vi "Test ARINC API.vi"() -> ()   [LabVIEW 2021]
doc: "ARINC API Tester."
uses:
  <vilib>/Utility/miscctls.llb/LVPointTypeDef.ctl
  <vilib>/Utility/error.llb/DialogType.ctl
  ARINC.lvlib
panel:
  in  "REQ Close Ref":bool
  out "Connect?":bool
  in  "serial number":u64
  in  "DAQ Type":enum16{"Hardware", "Simulation"}(ring)
  in  "REQ Initialize Hardware":bool
  in  "Show Diagram on Init":bool
  in  "Show Block Diagram":bool
  in  "Stop Module":bool
  in  "Start Module":bool
  in  "Hide Module Panel":bool
  in  "Show Module Panel":bool
  out "Status":string
  out "Module Running?":bool
  # "This VI tests the API for the Module."
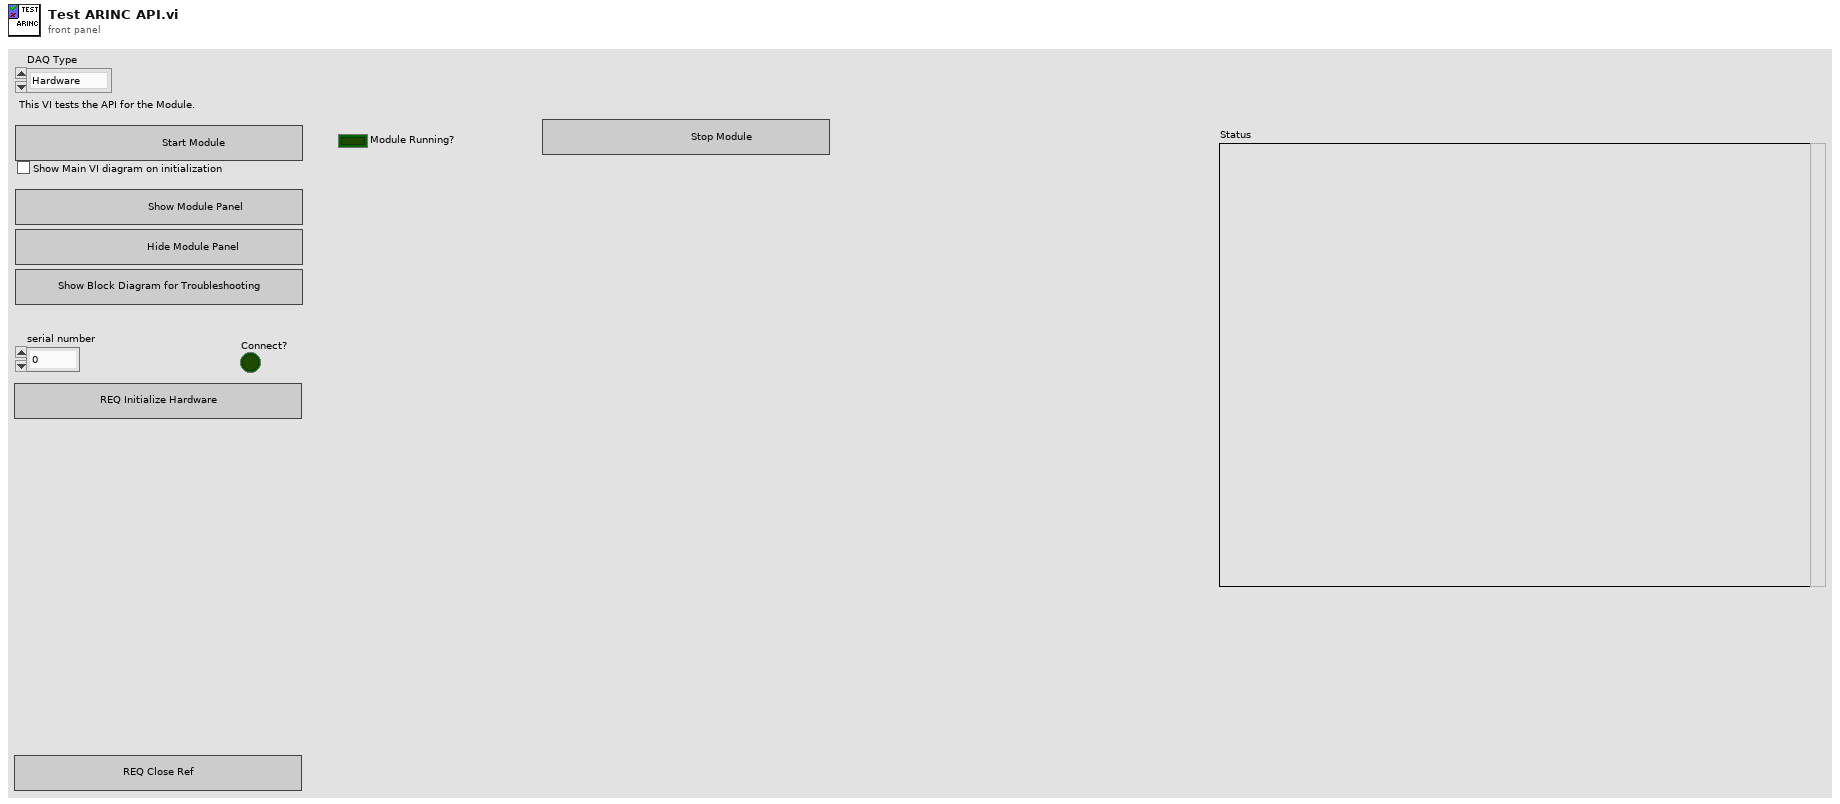
[diagram p1: front panel]
types:
  T1 = typedef "LVPointTypeDef.ctl" = cluster{"Horizontal":i16, "Vertical":i16}
  T2 = typedef "ARINC.lvlib/Broadcast Events--cluster.ctl" = cluster{"Module Did Init":refnum<user-event>, "Status Updated":refnum<user-event>, "Error Reported":refnum<user-event>, "Module Did Stop":refnum<user-event>, "Update Module Execution Status":refnum<user-event>}
  T3 = typedef "DialogType.ctl" = u16
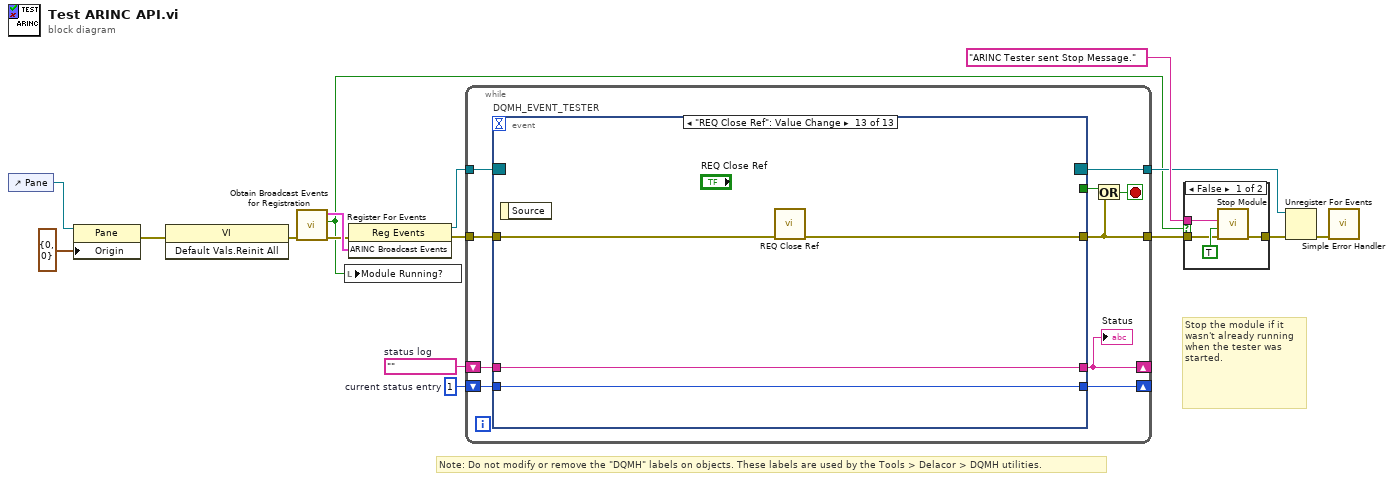
[diagram p0: block diagram]
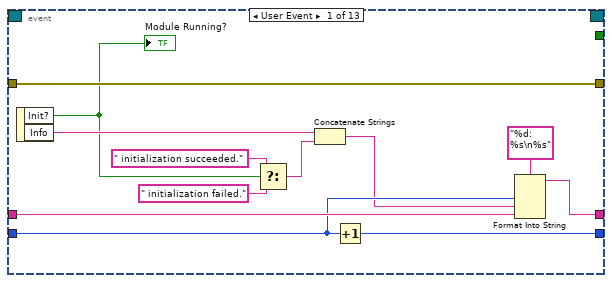
[diagram p3: hidden frame]
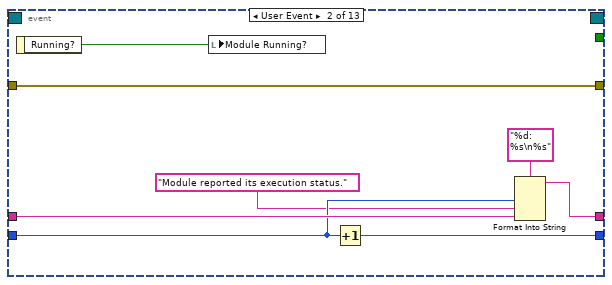
[diagram p4: hidden frame]
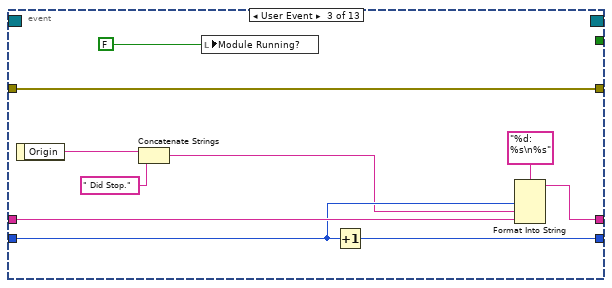
[diagram p5: hidden frame]
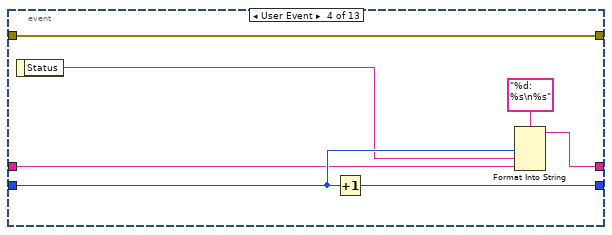
[diagram p6: hidden frame]
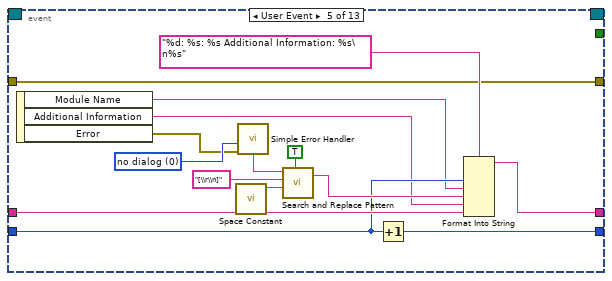
[diagram p7: hidden frame]
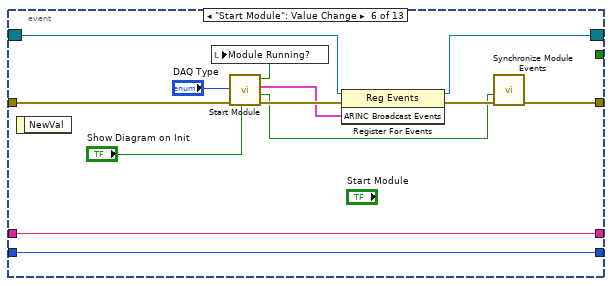
[diagram p8: hidden frame]
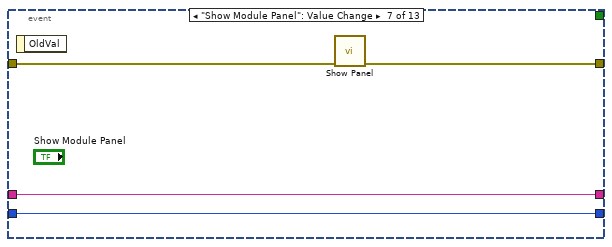
[diagram p9: hidden frame]
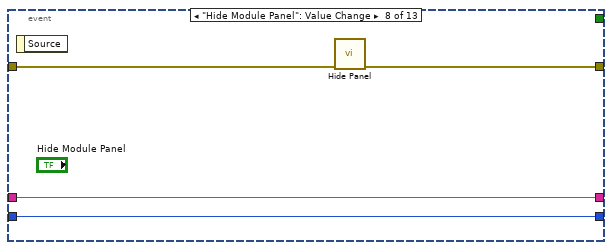
[diagram p10: hidden frame]
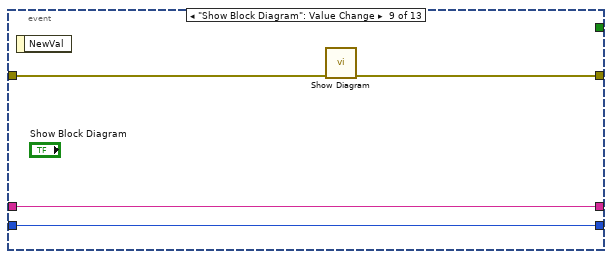
[diagram p11: hidden frame]
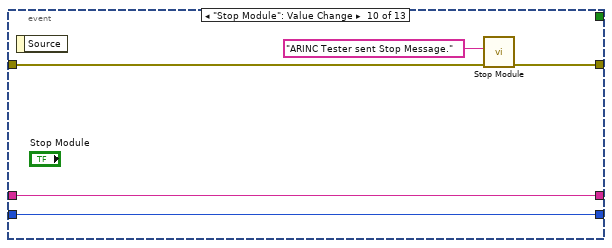
[diagram p12: hidden frame]
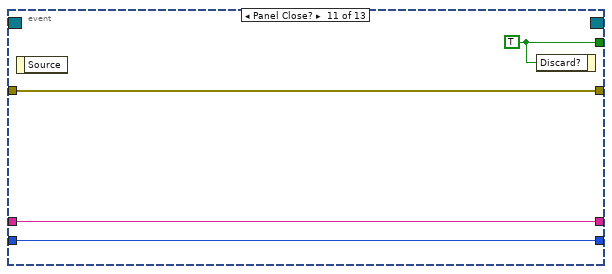
[diagram p13: hidden frame]
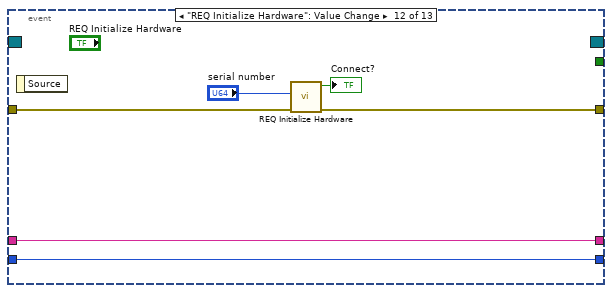
[diagram p14: hidden frame]
diagram:
  w13 = 1  # current status entry
  w14 = ""  # status log
  # "Stop the module if it wasn't already running when the tester was started."
  # "Note: Do not modify or remove the \"DQMH\" labels on objects. These labels are used by the Tools > Delacor > DQMH utilities."
  n1 = control-ref of="Pane"() -> (w2:refnum<vi>)
  n2 = property class="Pane"(reference=w2, "Origin"=T1 {"Horizontal"=0, "Vertical"=0}) -> (error out=w3:errorcluster)  [unwired: 1 in, 1 out]
  n3 = invoke class="VI" method="Default Vals.Reinit All"(error in=w3) -> (error out=w8:errorcluster)  [unwired: 2 in, 2 out]
  n4 = call "Obtain Broadcast Events for Registration.vi"("error in"=w8) -> ("error out"=w7:errorcluster, "Already running?"=w6:bool, "ARINC Broadcast Events"=w11:T2)  [unwired: 8 in]
  n5 = local write "Module Running?"(w6) -> ()
  n6 = register-events(error in=w7, w11) -> (reference out=w10:refnum<event-registration>, error out=w12:errorcluster)  [unwired: 1 in]
  n7 = while {
    tunnel: w10 -> [w26]
    tunnel: [w17] -> w5
    shift-right: [w21] -> _
    shift-left: w14 -> [w23]
    shift-right: [w22] -> _
    shift-left: w13 -> [w24]
    tunnel: w12 -> [w19]
    tunnel: [w18] -> w9
    stop <- w20 stop-if-true
    n8 = event "DQMH_EVENT_TESTER" shown="[12] \"REQ Close Ref\": Value Change" {
      selector: w26 -> [_ _ _ _ _ w85 _ _ _ _ _ _ _]
      dyn-events: [_ _ _ _ _ w84 _ _ _ _ _ _ _] -> w18
      timeout: _ -> [_ _ _ _ _ _ _ _ _ _ _ _ _]
      tunnel: [_ _ _ _ _ _ _ _ _ _ w112 _ _] -> w25
      tunnel: [w38 w40 w47 w57 w67 w83 w95 w99 w100 w106 w109 w115 w119] -> w17
      tunnel: w24 -> [w35 w44 w54 w60 w70 w88 w93 w97 w101 w107 w110 w116 w120]
      tunnel: w23 -> [w36 w45 w55 w59 w71 w89 w94 w98 w102 w108 w111 w117 w121]
      tunnel: [w33 w42 w52 w61 w69 w89 w94 w98 w102 w108 w111 w117 w121] -> w21
      tunnel: [w34 w43 w53 w63 w68 w88 w93 w97 w101 w107 w110 w116 w120] -> w22
      tunnel: w19 -> [w38 w40 w47 w57 w67 w82 w92 w96 w103 w104 w109 w118 w122]
      event User Event {
        n9 = event-data() -> ("Init?"=w30:bool, "Info"=w32:string)  [unwired: 1 in]
        "Module Running?" <- w30
        n10 = Select(t=" initialization succeeded.", s=w30, f=" initialization failed.") -> (s? t:f=w27:string)
        n11 = Concatenate Strings(w32, w27) -> (w31:string)
        n12 = Increment(x=w35) -> (x+1=w34:i32)
        n13 = Format Into String(format string="%d: %s\n%s", w35, w31, w36) -> (resulting string=w33:string)  [unwired: 2 in, 1 out]
      }
      event User Event {
        n14 = event-data() -> ("Running?"=w39:bool)  [unwired: 1 in]
        n15 = local write "Module Running?"(w39) -> ()
        n16 = Increment(x=w44) -> (x+1=w43:i32)
        n17 = Format Into String(format string="%d: %s\n%s", w44, "Module reported its execution status.", w45) -> (resulting string=w42:string)  [unwired: 2 in, 1 out]
      }
      event User Event {
        n18 = event-data() -> ("Origin"=w51:string)  [unwired: 1 in]
        n19 = Concatenate Strings(w51, " Did Stop.") -> (w50:string)
        n20 = local write "Module Running?"(FALSE ("Module Did Init?")) -> ()
        n21 = Increment(x=w54) -> (x+1=w53:i32)
        n22 = Format Into String(format string="%d: %s\n%s", w54, w50, w55) -> (resulting string=w52:string)  [unwired: 2 in, 1 out]
      }
      event User Event {
        n23 = event-data() -> ("Status"=w58:string)  [unwired: 1 in]
        n24 = Increment(x=w60) -> (x+1=w63:i32)
        n25 = Format Into String(format string="%d: %s\n%s", w60, w58, w59) -> (resulting string=w61:string)  [unwired: 2 in, 1 out]
      }
      event User Event {
        w72 = T3 0 items=["no dialog", "OK message", "continue or stop message", "OK message + warnings", "continue/stop + warnings"] ("type of dialog (OK msg:1)")
        n26 = event-data() -> ("Module Name"=w66:string, "Additional Information"=w65:string, "Error"=w64:errorcluster)  [unwired: 1 in]
        n27 = call <vilib>:"Space Constant.vi"() -> ("String"=w76:string)
        n28 = call <vilib>:"Simple Error Handler.vi"("type of dialog (OK msg:1)"=w72, "error in (no error)"=w64) -> ("message"=w73:string)  [unwired: 3 in, 4 out]
        n29 = call <vilib>:"Search and Replace Pattern.vi"("string"=w73, "regular expression (\"\")"="[\\r\\n]" ("regular expression (\"\")"), "replace string (\"\")"=w76, "replace all? (F)"=TRUE ("replace all CR/LF with spaces")) -> ("result string"=w74:string)  [unwired: 1 in, 1 out]
        n30 = Increment(x=w70) -> (x+1=w68:i32)
        n31 = Format Into String(format string="%d: %s: %s Additional Information: %s\n%s", w70, w66, w74, w65, w71) -> (resulting string=w69:string)  [unwired: 2 in, 1 out]
      }
      event "Start Module": Value Change {
        n32 = event-data() -> ()  [unwired: 1 in, 1 out]
        n33 = call "Start Module.vi"("Show Main VI Diagram on Init (F)"="Show Diagram on Init", "error in"=w82, "DAQ Type"="DAQ Type") -> ("error out"=w90:errorcluster, "Wait for Event Sync?"=w87:bool, "ARINC Broadcast Events"=w86:T2, "Module Was Already Running?"=w81:bool)  [unwired: 5 in]
        n34 = local write "Module Running?"(w81) -> ()
        n35 = register-events(reference=w85, error in=w90, w86) -> (reference out=w84:refnum<event-registration>, error out=w91:errorcluster)
        n36 = call "Synchronize Module Events.vi"("error in"=w91, "Wait for Event Sync?"=w87) -> ("error out"=w83:errorcluster)  [unwired: 9 in]
      }
      event "Show Module Panel": Value Change {
        n37 = event-data() -> ()  [unwired: 1 in, 1 out]
        n38 = call "Show Panel.vi"("error in (no error)"=w92) -> ("error out"=w95:errorcluster)  [unwired: 10 in]
      }
      event "Hide Module Panel": Value Change {
        n39 = event-data() -> ()  [unwired: 1 in, 1 out]
        n40 = call "Hide Panel.vi"("error in (no error)"=w96) -> ("error out"=w99:errorcluster)  [unwired: 10 in]
      }
      event "Show Block Diagram": Value Change {
        n41 = event-data() -> ()  [unwired: 1 in, 1 out]
        n42 = call "Show Diagram.vi"("error in (no error)"=w103) -> ("error out"=w100:errorcluster)  [unwired: 10 in]
      }
      event "Stop Module": Value Change {
        n43 = event-data() -> ()  [unwired: 1 in, 1 out]
        n44 = call "Stop Module.vi"("error in"=w104, "Origin"="ARINC Tester sent Stop Message.") -> ("error out"=w106:errorcluster)  [unwired: 9 in]
      }
      event Panel Close? {
        w112 = TRUE ("Discard?")
        n45 = event-data() -> ()  [unwired: 1 in, 1 out]
        n46 = event-data("Discard?"=w112) -> ()  [unwired: 1 in, 1 out]
      }
      event "REQ Initialize Hardware": Value Change {
        n47 = event-data() -> ()  [unwired: 1 in, 1 out]
        n48 = call "REQ Initialize Hardware.vi"("error in"=w118, "Connection Ref"="serial number") -> ("error out"=w115:errorcluster, "Connect?"=→"Connect?":bool)  [unwired: 7 in, 1 out]
      }
      event "REQ Close Ref": Value Change {
        n49 = event-data() -> ()  [unwired: 1 in, 1 out]
        n50 = call "REQ Close Ref.vi"("error in"=w122) -> ("error out"=w119:errorcluster)  [unwired: 10 in]
      }
    }
    "Status" <- w21
    n51 = Or(x=w25, y=w17) -> (x .or. y?=w20:bool)
  }
  n52 = case shown="False" w6 {
    tunnel: [w126 w127] -> w16
    tunnel: "ARINC Tester sent Stop Message." ("Origin") -> [w125 _]
    tunnel: w5 -> [w123 w127]
    frame False {
      n53 = call "Stop Module.vi"("error in"=w123, "Wait for Module to Stop? (F)"=TRUE ("Wait for Module to stop?"), "Origin"=w125) -> ("error out"=w126:errorcluster)  [unwired: 8 in]
    }
    frame True {
    }
  }
  n54 = Unregister For Events(event registration refnum=w9, error in=w16) -> (error out=w4:errorcluster)
  n55 = call <vilib>:"Simple Error Handler.vi"("error in (no error)"=w4) -> ()  [unwired: 4 in, 5 out]
